vi "TURCK GUI TestPanel RFID mehrer Module.vi"() -> ()   [LabVIEW 2017]
doc: "Example for reading and writing values for the TBEN-S2-2RFID-4DXP module from Turck"
uses:
  KH TURCK ETHERNETIP TDef Enum RFID Error.ctl
  KH TURCK ETHERNETIP TDefCluster TBEN-S2-2RFID-4DXP Status.ctl
  KH EthernetIPConfig 17.14/KH EthernetIPConfig TDef Config.ctl
  KH EthernetIPConfig 17.14/KH EthernetIPConfig TypeDefs ModuleTyp.ctl
  KH TURCK ETHERNETIP TDef Enum RFID Data RFID.ctl
  KH TURCK ETHERNETIP TDefCluster TURCK RFID.ctl
  KH TURCK ETHERNETIP TDef Enum RFID Act Command.ctl
  KH_DAQ 17.04/Turck/KH_DAQ_TURCK_TypeDefs_Cluster DI.ctl
  KH TURCK TypeDefs FGlob.ctl
  KH TURCK ETHERNETIP TDef Enum RFID User Command.ctl
  KH EthernetIP 17.19/KH_EthernetIP_Globals.vi
  KH_DAQ 17.04/Turck/KH_DAQ_TURCK_Global.vi
  KH TURCK ETHERNETIP RFID Global.vi
  KH TURCK ETHERNETIP Global.vi
panel:
  in  "EIP_DI":T1 {"Nr" max=63; "Chan" max=63}
  out "DI Modul2":bool[](array[boolean])
  out "DI Modul1":bool[](array[boolean])
  out "RFID 0 LS Array":T3[](array[typedef])
  in  "Write Kanal 1 Modul 2":u8[](array[numeric])
  in  "Write Kanal 0 Modul 2":u8[](array[numeric])
  in  "Write Kanal 1 Modul 1":u8[](array[numeric])
  in  "Write Kanal 0 Modul 1":u8[](array[numeric])
  out "RFID 0 Lesen Statemachine":T5[](array[typedef])
  out "Kanal 1 Modul 1":u8[](array[numeric])
  out "Kanal 1 Modul 2":u8[](array[numeric])
  out "Kanal 0 Modul 2":u8[](array[numeric])
  out "Kanal 0 Modul 1":u8[](array[numeric])
  out "UID Kanal 1 Modul 1":u8[](array[numeric])
  out "UID Kanal 1 Modul 2":u8[](array[numeric])
  out "UID Kanal 0 Modul2":u8[](array[numeric])
  out "UID Kanal 0 Modul 1":u8[](array[numeric])
  out "RFID 1 Lesen Statemachine":T5[](array[typedef])
  out "Error0 Modul 2":T6=33282
  out "Error1 Modul 2":T6=33282
  in  "Config":T7[](array[typedef])=[{"Typ"=enum."TBEN-S2-2RFID-4DXP", "Name"="1", "Nr."=1, "InputOutput"=[enum."Input", enum."Input", enum."Output", enum."Output"]}, {"Typ"=enum."TBEN-S2-2RFID-4DXP", "Name"="2", "Nr."=2, "InputOutput"=[enum."Output", enum."Output", enum."Input", enum."Input"]}]
  out "Status Array":T8[](array[typedef])=[{"Error writing 1"=FALSE, "ReadingFinished 1"=FALSE, "WritingFinished 1"=FALSE, "Error writing 0"=FALSE, "ReadingFinished 0"=FALSE, "WritingFinished 0"=FALSE, "Timeout 1"=FALSE, "State0"="Idle", "State1"="Start", "Timeout 0"=FALSE, "Successfull Writing 1"=FALSE, "Successfull Writing 0"=FALSE}, {"Error writing 1"=FALSE, "ReadingFinished 1"=FALSE, "WritingFinished 1"=FALSE, "Error writing 0"=FALSE, "ReadingFinished 0"=FALSE, "WritingFinished 0"=FALSE, "Timeout 1"=TRUE, "State0"="", "State1"="", "Timeout 0"=FALSE, "Successfull Writing 1"=FALSE, "Successfull Writing 0"=FALSE}]
  in  "Inventory":bool[](array[boolean])
  in  "Write":bool[](array[boolean])
  in  "Read":bool[](array[boolean])
  in  "Parameter RFID Array":T9(array[cluster])=[{"NumberOfBytes0"=312, "SizeFragmentRead1"=128, "SizeFragmentRead0"=128, "SizeFragmentWrite0"=128, "SizeFragmentWrite1"=128, "NumberOfBytes1"=312}, {"NumberOfBytes0"=312, "SizeFragmentRead1"=128, "SizeFragmentRead0"=128, "SizeFragmentWrite0"=128, "SizeFragmentWrite1"=128, "NumberOfBytes1"=312}]
  in  "TagNr":enum16{"Tag 0", "Tag 1"}(ring)
  out "Error1 Modul 1":T6=33282
  out "Error0 Modul 1":T6=33282
  in  "Reset message":bool caption="Button"
  in  "DOS":bool[](array[boolean])=[FALSE, FALSE, FALSE, FALSE, FALSE]
  out "error out":errorcluster
  in  "Exit":bool
  # "- Before starting the VI your PC has to be in the same subnet as the modules\n- Before starting the VI you have to the change the configuration. You have to change the operation mode into HF extended.\n- You have to set the number of bytes depending of the used tag"
  # "Kirschenhofer Maschinen GmbH\n\n\nRömerstraße 35, 89278 Nersingen-Straß\n\ninfo@kirschenhofer-gmbh.de"
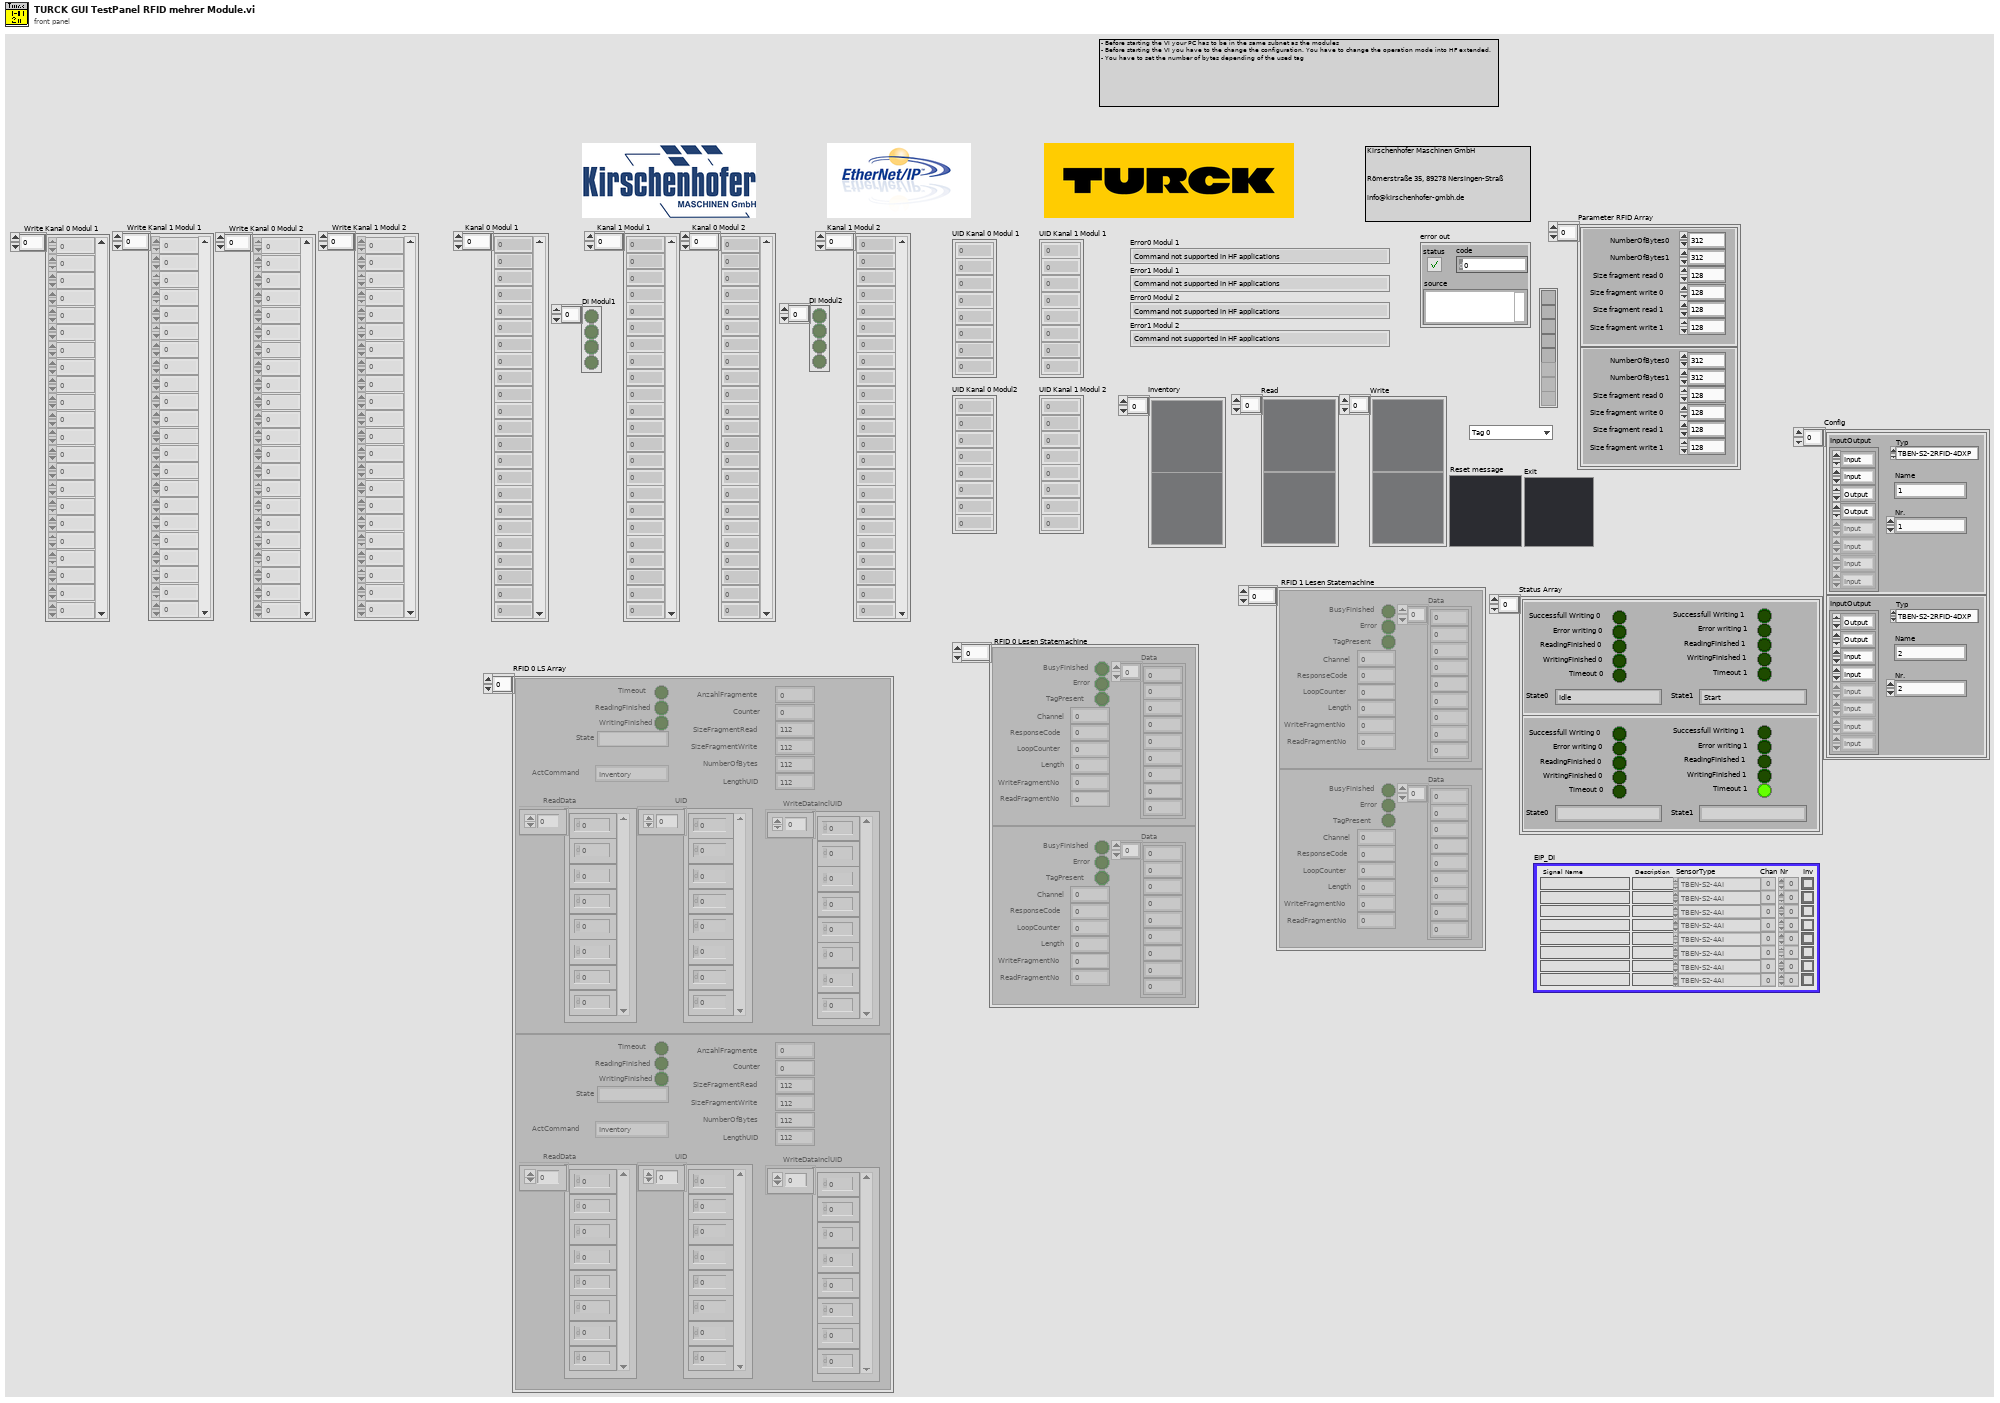
[diagram p1: front panel]
types:
  T1 = typedef "KH_DAQ_TURCK_TypeDefs_Cluster DI.ctl" = cluster{"Signal Name":string[], "Description":string[], "Chan":u16[], "Inv":bool[], "Nr":u16[], "SensorType":T2[]}
  T2 = typedef "KH EthernetIPConfig TypeDefs ModuleTyp.ctl" = enum16{"TBEN-S2-4AI", "TBEN-S1-8DXP", "TBEN-S2-2RFID-4DXP", "TBEN-S2-4AO", "TBEN-S2-4IOL"}
  T3 = typedef "KH TURCK ETHERNETIP TDefCluster TURCK RFID.ctl" = cluster{"NumberOfBytes":i32, "State":string, "Counter":i32, "ReadData":u8[], "AnzahlFragmente":i32, "WritingFinished":bool, "ReadingFinished":bool, "UID":u8[], "ActCommand":T4, "SizeFragmentRead":i32, "LengthUID":u16, "WriteDataInclUID":u8[], "Timeout":bool, "SizeFragmentWrite":i32}
  T4 = typedef "KH TURCK ETHERNETIP TDef Enum RFID Act Command.ctl" = enum16{"read", "write", "idle", "Inventory", ""}
  T5 = typedef "KH TURCK ETHERNETIP TDef Enum RFID Data RFID.ctl" = cluster{"ResponseCode":u16, "LoopCounter":u8, "Length":u16, "WriteFragmentNo":u8, "ReadFragmentNo":u8, "Data":u8[], "TagPresent":bool, "Error":bool, "BusyFinished":bool, "Channel":u16}
  T6 = typedef "KH TURCK ETHERNETIP TDef Enum RFID Error.ctl" = u16
  T7 = typedef "KH EthernetIPConfig TDef Config.ctl" = cluster{"Typ":T2, "Name":string, "Nr.":i32, "InputOutput":enum16{"Input", "Output"}[]}
  T8 = typedef "KH TURCK ETHERNETIP TDefCluster TBEN-S2-2RFID-4DXP Status.ctl" = cluster{"Error writing 1":bool, "ReadingFinished 1":bool, "WritingFinished 1":bool, "Error writing 0":bool, "ReadingFinished 0":bool, "WritingFinished 0":bool, "Timeout 1":bool, "State0":string, "State1":string, "Timeout 0":bool, "Successfull Writing 1":bool, "Successfull Writing 0":bool}
  T9 = cluster{"NumberOfBytes0":i32, "SizeFragmentRead1":i32, "SizeFragmentRead0":i32, "SizeFragmentWrite0":i32, "SizeFragmentWrite1":i32, "NumberOfBytes1":i32}[]
  T10 = typedef "KH TURCK TypeDefs FGlob.ctl" = enum16{"Put one", "Put all", "Recall one", "Recall all"}
  T11 = typedef "KH TURCK ETHERNETIP TDef Enum RFID User Command.ctl" = enum16{"read", "write", "idle", "inventory"}
  T12 = cluster{"TtoO NetworkConnID":u32, "OtoT NetworkConnID":u32, "OriginatorSerialNumber":u32, "ConnectionSerialNumber":u16}[]
  T13 = typedef "KH TURCK ETHERNETIP TDefCluster TBEN-S2-2RFID-4DXP Input Values.ctl" = cluster{"Station Status Word (Input Data Mapping)":cluster{"Module diagnostics avaliable":bool, "INFO: ARGEE Project Running":bool, "Undervoltage V2":bool, "Undervoltage V1":bool, "Internal Error":bool, "I/O-ASSISTANT Force Mode active":bool}, "RFID control/status 0 (Input Data Mapping)":cluster{"Tag present at r/w head":bool[], "response code":u16, "loop counter":u8, "Length":u16, "Error code":u16, "Tag counter":u16, "Data (Bytes) available":u16, "Read fragment No.":u8, "Write fragment No.":u8, "Tag present at r/w head bit":bool, "HF r/w head switched on":bool, "Continuous mode active":bool, "Antenna detuned at HF read/write head":bool, "Parameter not supported by read/write head":bool, "Error reported by read/write head":bool, "Not connected to read/write head":bool}, "RFID read data 0 (Input Data Mapping)":u8[], "RFID control/status 1 (Input Data Mapping)":cluster{"response code":u16, "Loop counter":u8, "Length":u16, "Error code":u16, "Tag counter":u16, "Data (Bytes) available":u16, "Read fragment No.":u8, "Write fragment No.":u8, "Tag present at r/w head bit":bool, "HF r/w head switched on":bool, "Continuous mode active":bool, "Antenna detuned at HF read/write head":bool, "Parameter not supported by read/write head":bool, "Error reported by read/write head":bool, "Not connected to read/write head":bool, "Tag present at r/w head":bool[]}, "RFID read data 1 (Input Data Mapping)":u8[], "RFID diagnostics (Input Data Mapping)":cluster{"Overcurrent supply VAUX1 (a)":bool, "Parameterization error (a)":bool, "Configuration via DTM active (a)":bool, "Buffer full (a)":bool, "Antenna detuned at HF read/write head (a)":bool[], "Parameter not supported by read/write head (a)":bool[], "Error reported by read/write head (a)":bool[], "Not connected to read/write head (a)":bool[], "Overcurrent supply VAUX1 (b)":bool, "Parameterization error (b)":bool, "Configuration via DTM active (b)":bool, "Buffer full (b)":bool, "Antenna detuned at HF read/write head (b)":bool[], "Parameter not supported by read/write head (b)":bool[], "Error reported by read/write head (b)":bool[], "Not connected to read/write head (b)":bool[]}, "DXP diagnostics (Input Data Mapping)":cluster{"Overcurrent VAUX2 Ch4/5":bool, "Overcurrent VAUX2 Ch6/7":bool, "Channel 4 - Output overcurrent":bool, "Channel 5 - Output overcurrent":bool, "Channel 6 - Output overcurrent":bool, "Channel 7 - Output overcurrent":bool}, "DXP (Input Data Mapping)":cluster{"Channel 4 - Input value":bool, "Channel 5 - Input value":bool, "Channel 6 - Input value":bool, "Channel 7 - Input value":bool}}
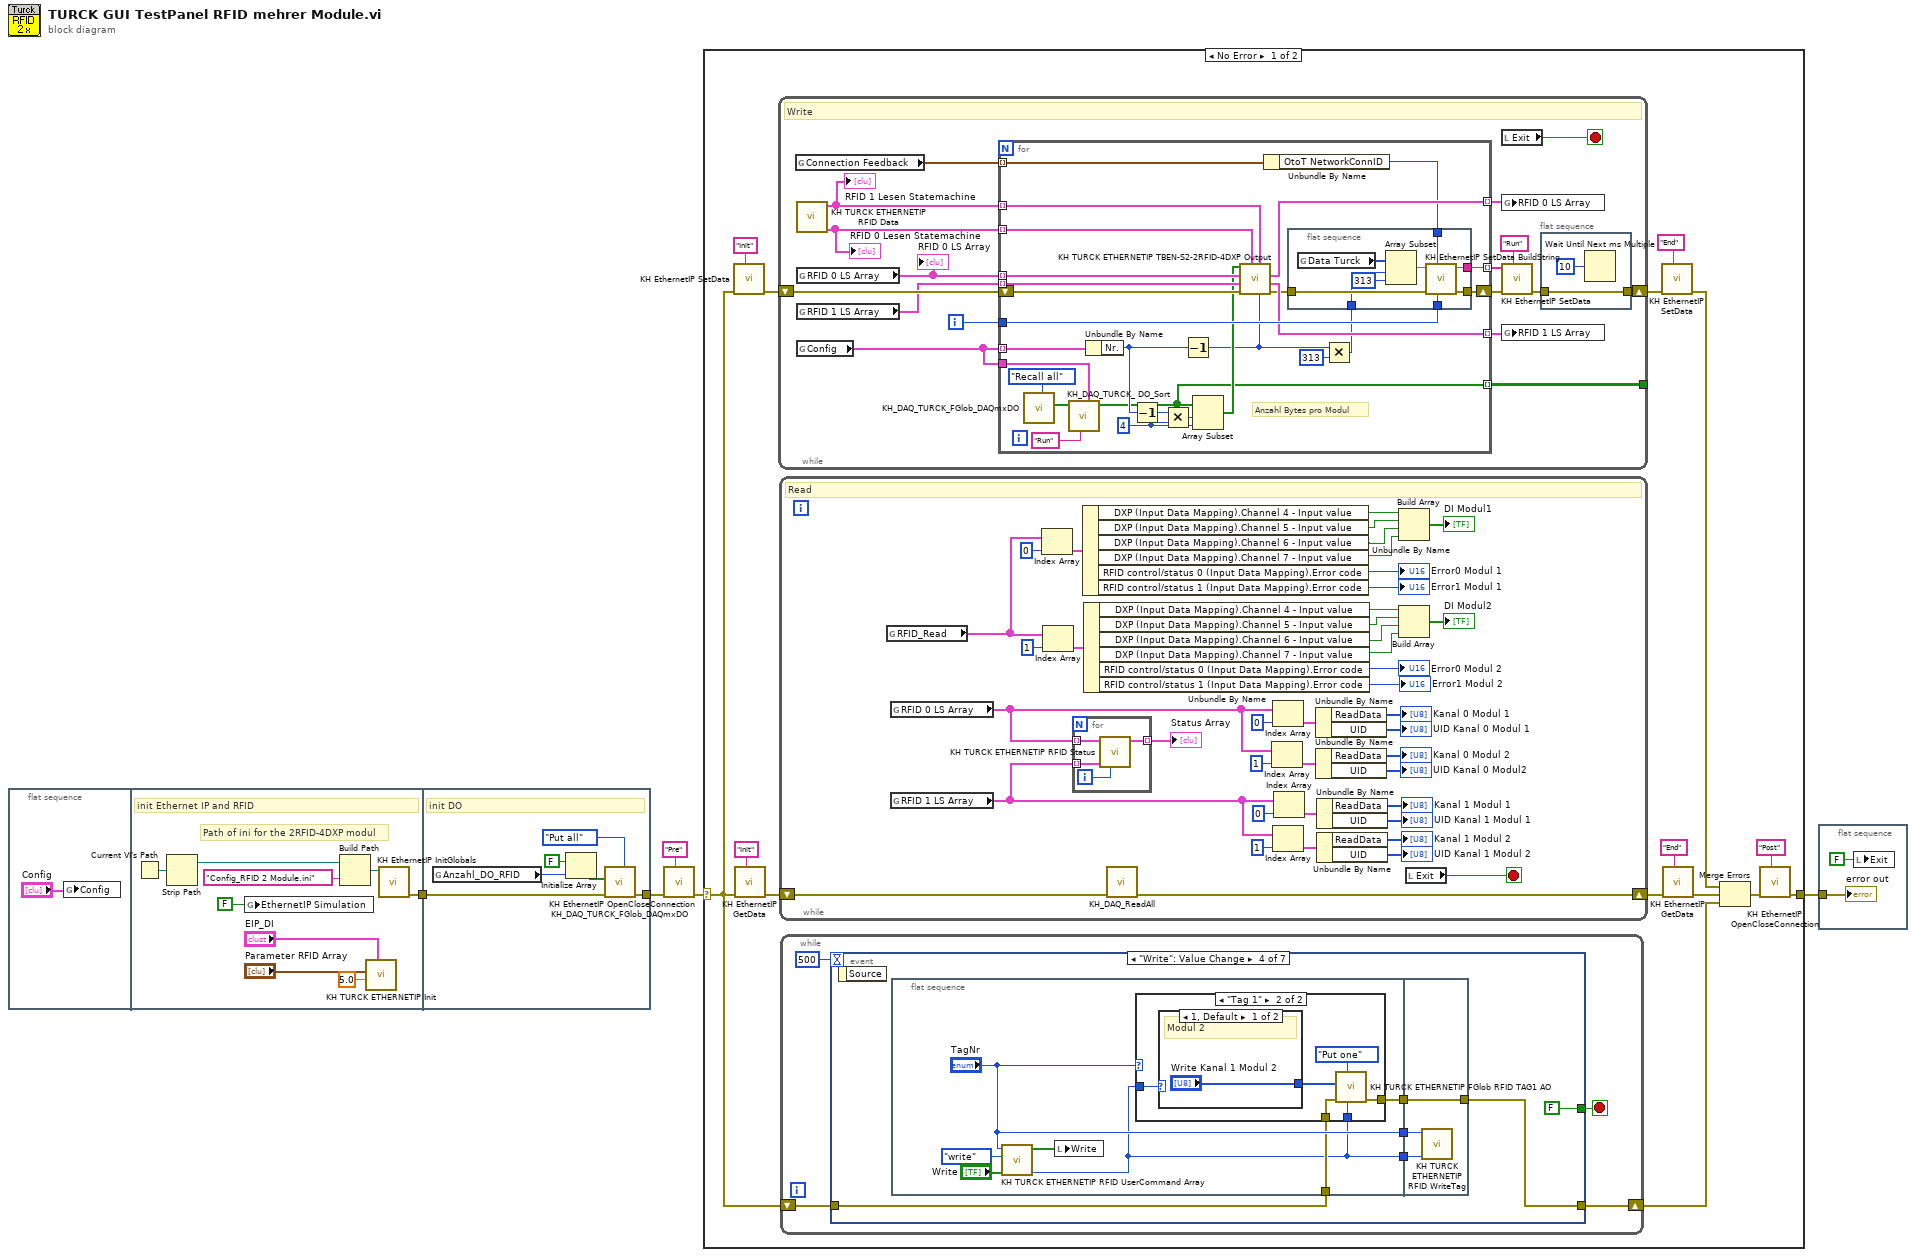
[diagram p0: block diagram]
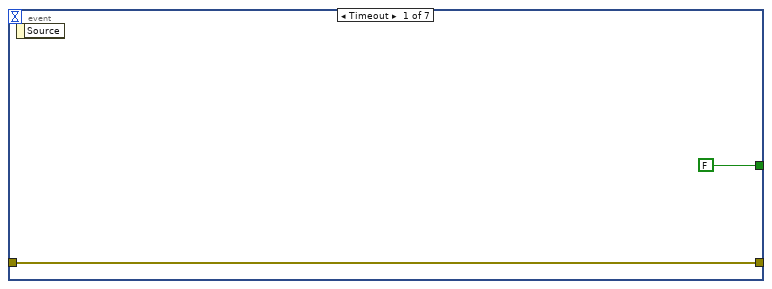
[diagram p2: hidden frame]
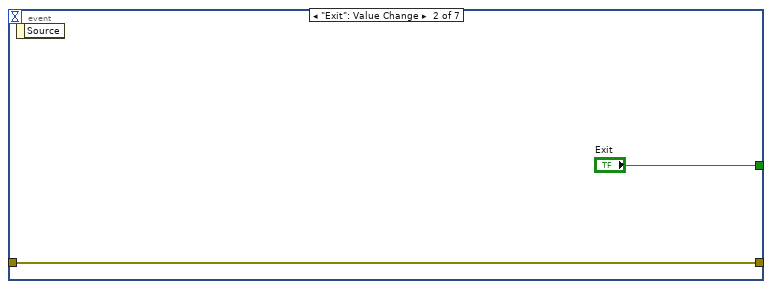
[diagram p3: hidden frame]
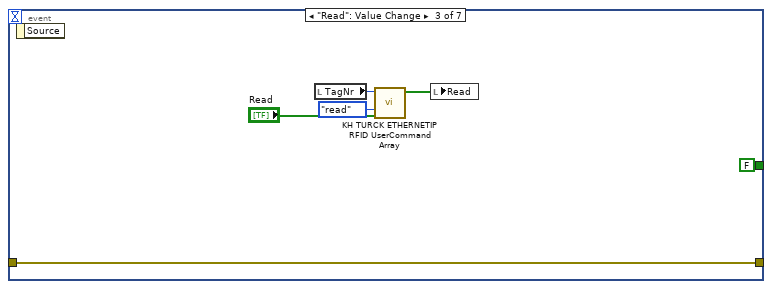
[diagram p4: hidden frame]
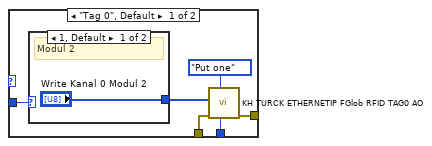
[diagram p5: hidden frame]
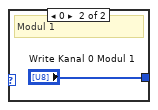
[diagram p6: hidden frame]
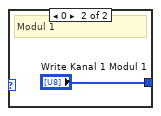
[diagram p7: hidden frame]
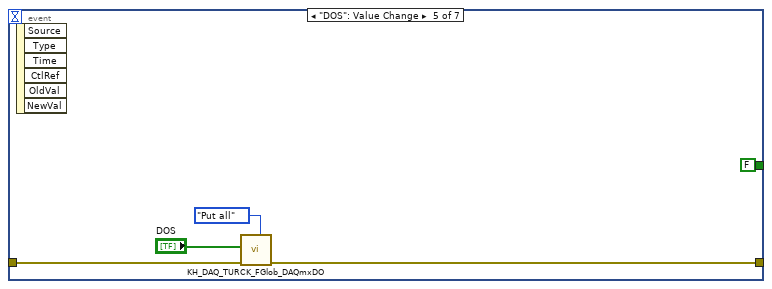
[diagram p8: hidden frame]
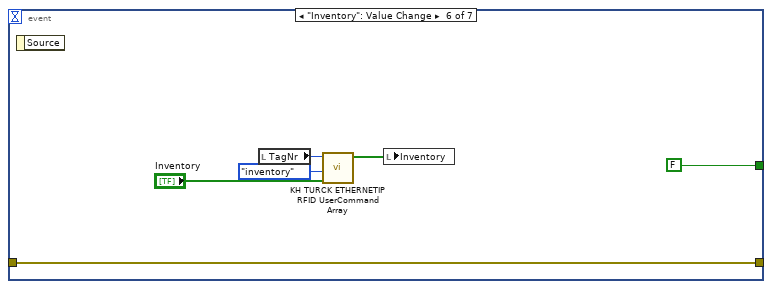
[diagram p9: hidden frame]
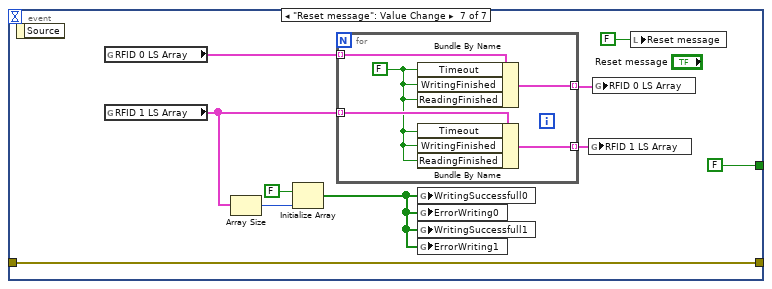
[diagram p10: hidden frame]
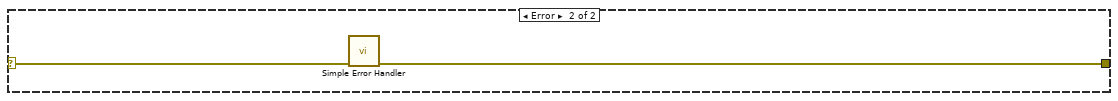
[diagram p11: hidden frame]
diagram:
  n1 = flat-sequence {
    tunnel: [w11] -> w1
    tunnel: [w17] -> w3
    tunnel: w1 -> [w16]
    frame #0 {
      n2 = global write "KH_EthernetIP_Globals.vi" "Config"("Config") -> ()
    }
    frame #1 {
      # "Path of ini for the 2RFID-4DXP modul"
      # "init Ethernet IP and RFID"
      n3 = Current VI's Path() -> (path=w15:path)
      n4 = Strip Path(path=w15) -> (stripped path=w14:path)  [unwired: 1 out]
      n5 = global write "KH_EthernetIP_Globals.vi" "EthernetIP Simulation"(FALSE ("EthernetIP Simulation")) -> ()
      n6 = Build Path(base path=w14, name or relative path="Config_RFID 2 Module.ini") -> (appended path=w12:path)
      n7 = call "KH TURCK ETHERNETIP Init.vi"("EIP_DI"="EIP_DI", "TimeoutRFID"=5.0 ("Timeout"), "Parameter RFID Array"="Parameter RFID Array") -> ()  [unwired: 8 in, 1 out]
      n8 = call "KH EthernetIP InitGlobals.vi"("Config File"=w12) -> ("err out"=w11:errorcluster)  [unwired: 10 in]
    }
    frame #2 {
      # "init DO"
      n9 = global read "KH_DAQ_TURCK_Global.vi" "Anzahl_DO_RFID"() -> (w20:i32)
      n10 = Initialize Array(FALSE ("values"), w20) -> (w18:bool[])
      n11 = call "KH_DAQ_TURCK_FGlob_DAQmxDO.vi"("Function (Recall One)"=KH_TURCK_TypeDefs_FGlob."Put all" ("Function"), "err in"=w16, "DXP Values IN"=w18) -> ("err out"=w17:errorcluster)  [unwired: 5 in, 3 out]
    }
  }
  n12 = call "KH EthernetIP OpenCloseConnection.vi"("Function"="Pre", "error in"=w3) -> ("error out"=w4:errorcluster)  [unwired: 9 in]
  n13 = case shown="No Error" w4 {
    selector: w4 -> [w22 w210]
    tunnel: [w23 w209] -> w2
    frame No Error {
      n14 = call "KH EthernetIP SetData.vi"("Function"="Init", "error in"=w22) -> ("error out"=w26:errorcluster)  [unwired: 7 in, 2 out]
      n15 = call "KH EthernetIP GetData.vi"("Function"="Init", "error in"=w22) -> ("error out"=w36:errorcluster)  [unwired: 8 in, 1 out]
      n16 = while {
        shift-right: [w51] -> w27
        shift-left: w26 -> [w49]
        tunnel: [w37] -> _
        i -> [w48]
        stop <- w47 stop-if-true
        # "Write"
        n17 = global read "KH_EthernetIP_Globals.vi" "Connection Feedback"() -> (w41:T12)
        n18 = call "KH TURCK ETHERNETIP RFID Data.vi"() -> ("RFID 0 Read SM"=w39:T5[], "RFID 1 Read SM"=w40:T5[])  [unwired: 10 in]
        "RFID 1 Lesen Statemachine" <- w40
        "RFID 0 Lesen Statemachine" <- w39
        n19 = global read "KH TURCK ETHERNETIP RFID Global.vi" "RFID 0 LS Array"() -> (w43:T3[])
        "RFID 0 LS Array" <- w43
        n20 = global read "KH TURCK ETHERNETIP RFID Global.vi" "RFID 1 LS Array"() -> (w45:T3[])
        n21 = global read "KH_EthernetIP_Globals.vi" "Config"() -> (w38:T7[])
        n22 = for {
          tunnel: [w79] -> w46 mode=indexing
          tunnel: w48 -> [w77]
          shift-right: [w80] -> w50
          shift-left: w49 -> [w78]
          tunnel: w40 -> [w66] mode=indexing
          tunnel: w39 -> [w67] mode=indexing
          tunnel: w43 -> [w74] mode=indexing
          tunnel: w45 -> [w76] mode=indexing
          tunnel: [w75] -> w44 mode=indexing
          tunnel: [w73] -> w42 mode=indexing
          tunnel: w38 -> [w58] mode=indexing
          tunnel: w41 -> [w69] mode=indexing
          tunnel: w38 -> [w57]
          tunnel: [w56] -> w37 mode=indexing
          w59 = 4 ("length")
          # "Anzahl Bytes pro Modul"
          n23 = call "KH_DAQ_TURCK_FGlob_DAQmxDO.vi"("Function (Recall One)"=KH_TURCK_TypeDefs_FGlob."Recall all") -> ("DXP Values OUT"=w63:bool[])  [unwired: 7 in, 3 out]
          n24 = call "KH_DAQ_TURCK_ DO_Sort.vi"("Config"=w57, "Function"="Run", "DOs"=w63) -> ("DO_RFID"=w56:bool[])  [unwired: 5 in, 3 out]
          n25 = Unbundle By Name(w58) -> ("Nr."=w64:i32)
          n26 = Decrement(x=w64) -> (x-1=w60:i32)
          n27 = Multiply(x=w60, y=w59) -> (x*y=w61:i32)
          n28 = Decrement(x=w64) -> (x-1=w55:i32)
          n29 = Array Subset(array=w56, index=w61, length=w59) -> (w62:bool[])
          n30 = call "KH TURCK ETHERNETIP TBEN-S2-2RFID-4DXP Output.vi"("Nr Modul"=w55, "Read 1 SM"=w66, "Read 0 SM"=w67, "error in"=w78, "ReadWrite 1 SM In"=w76, "ReadWrite 0 SM In"=w74, "RFID DXP"=w62) -> ("error out"=w72:errorcluster, "ReadWrite 1 SM Out"=w75:T3, "ReadWrite 0 SM Out"=w73:T3)  [unwired: 1 in, 1 out]
          n31 = Unbundle By Name(w69) -> ("OtoT NetworkConnID"=w68:u32)
          n32 = flat-sequence {
            tunnel: [w89] -> w80
            tunnel: w68 -> [w88]
            tunnel: [w87] -> w79
            tunnel: w77 -> [w86]
            tunnel: w72 -> [w84]
            tunnel: w71 -> [w83]
            frame #0 {
              n33 = global read "KH TURCK ETHERNETIP Global.vi" "Data Turck"() -> (w81:u8[])
              n34 = Array Subset(array=w81, index=w83, length=313) -> (w82:u8[])
              n35 = call "KH EthernetIP SetData BuildString.vi"("LoopIndex"=w86, "OtoT NetworkConnID"=w88, "error in"=w84, "Output Data"=w82) -> ("error out"=w89:errorcluster, "DataString"=w87:string)  [unwired: 6 in]
            }
          }
          n36 = Multiply(x=w55, y=313) -> (x*y=w71:i32)
        }
        n37 = local read "Exit"() -> (w47:bool)
        n38 = global write "KH TURCK ETHERNETIP RFID Global.vi" "RFID 0 LS Array"(w42) -> ()
        n39 = call "KH EthernetIP SetData.vi"("Function"="Run", "error in"=w50, "Data Strings"=w46) -> ("error out"=w52:errorcluster)  [unwired: 6 in, 2 out]
        n40 = global write "KH TURCK ETHERNETIP RFID Global.vi" "RFID 1 LS Array"(w44) -> ()
        n41 = flat-sequence {
          tunnel: w52 -> [w90]
          tunnel: [w90] -> w51
          frame #0 {
            n42 = Wait Until Next ms Multiple(millisecond multiple=u32 10) -> ()  [unwired: 1 out]
          }
        }
      }
      n43 = while {
        shift-right: [w92] -> w34
        shift-left: w36 -> [w132]
        stop <- w128 stop-if-true
        # "Read"
        n44 = global read "KH TURCK ETHERNETIP Global.vi" "RFID_Read"() -> (w93:T13[])
        n45 = global read "KH TURCK ETHERNETIP RFID Global.vi" "RFID 0 LS Array"() -> (w117:T3[])
        n46 = global read "KH TURCK ETHERNETIP RFID Global.vi" "RFID 1 LS Array"() -> (w108:T3[])
        n47 = Index Array(array=w93, index=0) -> (element=w124:T13)
        n48 = Index Array(array=w93, index=1) -> (element=w102:T13)
        n49 = for {
          tunnel: w117 -> [w136] mode=indexing
          tunnel: w108 -> [w135] mode=indexing
          tunnel: [w134] -> w127 mode=indexing
          i -> [w133]
          n50 = call "KH TURCK ETHERNETIP RFID Status.vi"("Nr.Module"=w133, "RFID 1"=w135, "RFID 0"=w136) -> ("StatusOUT"=w134:T8)  [unwired: 8 in]
        }
        "Status Array" <- w127
        n51 = Unbundle By Name(w124) -> ("DXP (Input Data Mapping).Channel 4 - Input value"=w107:bool, "DXP (Input Data Mapping).Channel 5 - Input value"=w106:bool, "DXP (Input Data Mapping).Channel 6 - Input value"=w105:bool, "DXP (Input Data Mapping).Channel 7 - Input value"=w104:bool, "RFID control/status 0 (Input Data Mapping).Error code"=→"Error0 Modul 1":u16, "RFID control/status 1 (Input Data Mapping).Error code"=→"Error1 Modul 1":u16)
        n52 = Unbundle By Name(w102) -> ("DXP (Input Data Mapping).Channel 4 - Input value"=w97:bool, "DXP (Input Data Mapping).Channel 5 - Input value"=w96:bool, "DXP (Input Data Mapping).Channel 6 - Input value"=w95:bool, "DXP (Input Data Mapping).Channel 7 - Input value"=w94:bool, "RFID control/status 0 (Input Data Mapping).Error code"=→"Error0 Modul 2":u16, "RFID control/status 1 (Input Data Mapping).Error code"=→"Error1 Modul 2":u16)
        n53 = call "KH_DAQ_ReadAll.vi"("err in"=w132) -> ("err out"=w92:errorcluster)  [unwired: 10 in]
        n54 = Index Array(array=w117, index=1) -> (element=w120:T3)
        n55 = Index Array(array=w117, index=0) -> (element=w125:T3)
        n56 = Index Array(array=w108, index=1) -> (element=w114:T3)
        n57 = Index Array(array=w108, index=0) -> (element=w111:T3)
        n58 = Unbundle By Name(w125) -> ("ReadData"=→"Kanal 0 Modul 1":u8[], "UID"=→"UID Kanal 0 Modul 1":u8[])
        n59 = Unbundle By Name(w120) -> ("ReadData"=→"Kanal 0 Modul 2":u8[], "UID"=→"UID Kanal 0 Modul2":u8[])
        n60 = Unbundle By Name(w111) -> ("ReadData"=→"Kanal 1 Modul 1":u8[], "UID"=→"UID Kanal 1 Modul 1":u8[])
        n61 = Unbundle By Name(w114) -> ("ReadData"=→"Kanal 1 Modul 2":u8[], "UID"=→"UID Kanal 1 Modul 2":u8[])
        n62 = Build Array(w107, w106, w105, w104) -> (→"DI Modul1":bool[])
        n63 = Build Array(w97, w96, w95, w94) -> (→"DI Modul2":bool[])
        n64 = local read "Exit"() -> (w128:bool)
      }
      n65 = while {
        shift-right: [w137] -> w24
        shift-left: w22 -> [w139]
        stop <- w140 stop-if-true
        n66 = event shown="[3] \"Write\": Value Change" {
          selector: _ -> [_ _ _ _ _ _ _]
          dyn-events: _ -> [_ _ _ _ _ _ _]
          timeout: 500 -> [_ _ _ _ _ _ _]
          tunnel: [FALSE ("Exit") "Exit" FALSE ("Exit") FALSE ("Exit") FALSE ("Exit") FALSE ("Exit") FALSE ("Exit")] -> w140
          tunnel: w139 -> [w141 w143 w149 w155 w185 w192 w202]
          tunnel: [w141 w143 w149 w154 w184 w192 w202] -> w137
          event Timeout {
            n67 = event-data() -> ()  [unwired: 1 in, 1 out]
          }
          event "Exit": Value Change {
            n68 = event-data() -> ()  [unwired: 1 in, 1 out]
          }
          event "Read": Value Change {
            n69 = event-data() -> ()  [unwired: 1 in, 1 out]
            n70 = local read "TagNr"() -> (w148:enum16{"Tag 0", "Tag 1"})
            n71 = call "KH TURCK ETHERNETIP RFID UserCommand Array.vi"("BitArray"="Read", "UserCommand"=KH_TURCK_ETHERNETIP_TDef_Enum_RFID_User_Command."read", "TagNr"=w148) -> ("initialized array"=w145:bool[])  [unwired: 7 in, 1 out]
            n72 = local write "Read"(w145) -> ()
          }
          event "Write": Value Change {
            n73 = event-data() -> ()  [unwired: 1 in, 1 out]
            n74 = flat-sequence {
              tunnel: w155 -> [w158]
              tunnel: [w159] -> w153
              tunnel: ["TagNr"] -> w152
              tunnel: [w157] -> w151
              tunnel: [w182] -> w154
              tunnel: w153 -> [w182]
              tunnel: w152 -> [w181]
              tunnel: w151 -> [w180]
              frame #0 {
                n75 = call "KH TURCK ETHERNETIP RFID UserCommand Array.vi"("BitArray"="Write", "UserCommand"=KH_TURCK_ETHERNETIP_TDef_Enum_RFID_User_Command."write", "TagNr"="TagNr") -> ("index of element"=w157:i32, "initialized array"=w161:bool[])  [unwired: 7 in]
                n76 = local write "Write"(w161) -> ()
                n77 = case shown="\"Tag 1\"" "TagNr" {
                  tunnel: w157 -> [w169 w177]
                  tunnel: [w166 w176] -> w159
                  tunnel: w158 -> [w165 w175]
                  tunnel: w157 -> [w164 w172]
                  frame "Tag 0", Default {
                    n78 = case shown="1, Default" w169 {
                      tunnel: ["Write Kanal 0 Modul 2" "Write Kanal 0 Modul 1"] -> w168
                      frame 1, Default {
                        # "Modul 2"
                      }
                      frame 0 {
                        # "Modul 1"
                      }
                    }
                    n79 = call "KH TURCK ETHERNETIP FGlob RFID TAG0 AO.vi"("Nr Module"=w164, "Function"=KH_TURCK_TypeDefs_FGlob."Put one", "err in"=w165, "RFID one in"=w168) -> ("err out"=w166:errorcluster)  [unwired: 5 in, 2 out]
                  }
                  frame "Tag 1" {
                    n80 = case shown="1, Default" w177 {
                      tunnel: ["Write Kanal 1 Modul 2" "Write Kanal 1 Modul 1"] -> w173
                      frame 1, Default {
                        # "Modul 2"
                      }
                      frame 0 {
                        # "Modul 1"
                      }
                    }
                    n81 = call "KH TURCK ETHERNETIP FGlob RFID TAG1 AO.vi"("Nr Module"=w172, "Function"=KH_TURCK_TypeDefs_FGlob."Put one", "err in"=w175, "RFID one in"=w173) -> ("err out"=w176:errorcluster)  [unwired: 5 in, 2 out]
                  }
                }
              }
              frame #1 {
                n82 = call "KH TURCK ETHERNETIP RFID WriteTag.vi"("Modul Nr"=w180, "TagNr"=w181) -> ()  [unwired: 10 in]
              }
            }
          }
          event "DOS": Value Change {
            n83 = event-data() -> ()  [unwired: 1 in, 6 out]
            n84 = call "KH_DAQ_TURCK_FGlob_DAQmxDO.vi"("Function (Recall One)"=KH_TURCK_TypeDefs_FGlob."Put all", "err in"=w185, "DXP Values IN"="DOS") -> ("err out"=w184:errorcluster)  [unwired: 5 in, 3 out]
          }
          event "Inventory": Value Change {
            n85 = event-data() -> ()  [unwired: 1 in, 1 out]
            n86 = local read "TagNr"() -> (w191:enum16{"Tag 0", "Tag 1"})
            n87 = call "KH TURCK ETHERNETIP RFID UserCommand Array.vi"("BitArray"="Inventory", "UserCommand"=KH_TURCK_ETHERNETIP_TDef_Enum_RFID_User_Command."inventory", "TagNr"=w191) -> ("initialized array"=w188:bool[])  [unwired: 7 in, 1 out]
            n88 = local write "Inventory"(w188) -> ()
          }
          event "Reset message": Value Change {
            n89 = event-data() -> ()  [unwired: 1 in, 1 out]
            n90 = global read "KH TURCK ETHERNETIP RFID Global.vi" "RFID 0 LS Array"() -> (w199:T3[])
            n91 = global read "KH TURCK ETHERNETIP RFID Global.vi" "RFID 1 LS Array"() -> (w194:T3[])
            n92 = Array Size(array=w194) -> (size(s)=w198:i32)
            n93 = Initialize Array(FALSE ("TimeoutReading"), w198) -> (w195:bool[])
            n94 = for {
              tunnel: [w208] -> w200 mode=indexing
              tunnel: w199 -> [w207] mode=indexing
              tunnel: [w206] -> w196 mode=indexing
              tunnel: w194 -> [w205] mode=indexing
              w204 = FALSE ("TimeoutReading")
              n95 = Bundle By Name(cluster=w207, "Timeout"=w204, "WritingFinished"=w204, "ReadingFinished"=w204) -> (w208:T3)
              n96 = Bundle By Name(cluster=w205, "Timeout"=w204, "WritingFinished"=w204, "ReadingFinished"=w204) -> (w206:T3)
            }
            n97 = global write "KH TURCK ETHERNETIP RFID Global.vi" "WritingSuccessfull0"(w195) -> ()
            n98 = global write "KH TURCK ETHERNETIP RFID Global.vi" "ErrorWriting0"(w195) -> ()
            n99 = global write "KH TURCK ETHERNETIP RFID Global.vi" "WritingSuccessfull1"(w195) -> ()
            n100 = global write "KH TURCK ETHERNETIP RFID Global.vi" "ErrorWriting1"(w195) -> ()
            n101 = global write "KH TURCK ETHERNETIP RFID Global.vi" "RFID 1 LS Array"(w196) -> ()
            n102 = global write "KH TURCK ETHERNETIP RFID Global.vi" "RFID 0 LS Array"(w200) -> ()
            n103 = local write "Reset message"(FALSE ("TimeoutWriting")) -> ()
          }
        }
      }
      n104 = call "KH EthernetIP SetData.vi"("Function"="End", "error in"=w27) -> ("error out"=w31:errorcluster)  [unwired: 7 in, 2 out]
      n105 = call "KH EthernetIP GetData.vi"("Function"="End", "error in"=w34) -> ("error out"=w29:errorcluster)  [unwired: 8 in, 1 out]
      n106 = Merge Errors(w31, w29, w24) -> (w30:errorcluster)
      n107 = call "KH EthernetIP OpenCloseConnection.vi"("Function"="Post", "error in"=w30) -> ("error out"=w23:errorcluster)  [unwired: 9 in]
    }
    frame Error {
      n108 = call <vilib>:"Simple Error Handler.vi"("error in (no error)"=w210) -> ("error out"=w209:errorcluster)  [unwired: 4 in, 4 out]
    }
  }
  n109 = flat-sequence {
    tunnel: w2 -> [w211]
    frame #0 {
      n110 = local write "Exit"(FALSE ("Exit")) -> ()
      "error out" <- w211
    }
  }
